vi "ADS Des TCV.vi"(8 "error in (no error)":errorcluster, 11 "ref in":u64) -> (0 "error out":errorcluster)   [LabVIEW 2024]
uses:
  TransformCV-LabVIEW/Test/dependencies_dll_release/TCV_Lib.dll
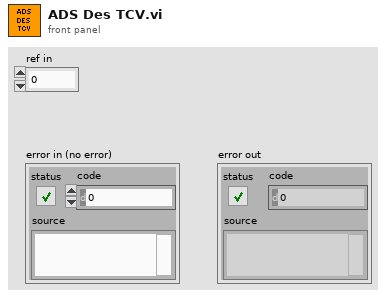
[diagram p1: front panel]
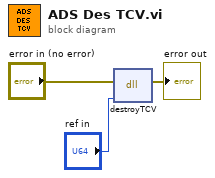
[diagram p0: block diagram]
diagram:
  n1 = dll-call lib="D:/TransformCV-LabVIEW/Test/dependencies_dll_release/TCV_Lib.dll" fn="destroyTCV"(error in="error in (no error)", "ref in"="ref in") -> (error out=→"error out":errorcluster)  [unwired: 4 in, 1 out]
